vi "remote.Read Dev.Modules.vi"(8 "error in (no error)":errorcluster, 11 "SLSC Remote in":refnum<class "SLSC Interface.lvclass">) -> (0 "error out":errorcluster, 2 "Dev.Modules":refnum<k21>[](array[refnum]), 3 "SLSC Remote out":refnum<class "SLSC Interface.lvclass">)   [LabVIEW 2016, in "SLSC Interface.lvclass"]
uses:
  SLSC Interface Class/SLSC Interface.lvclass
  <vilib>/NI/JSON Support for LabVIEW/JSON Data Classes/JSON Helper/To More Specific Type (Array).vi
  <vilib>/NI/JSON Support for LabVIEW/JSON Data Classes/JSON Array/Index Array (String Value).vi
  <vilib>/NI/JSON Support for LabVIEW/JSON Data Classes/JSON Helper/JSON Helper.lvclass
  <vilib>/NI/JSON Support for LabVIEW/JSON Data Classes/JSON Array/JSON Array.lvclass
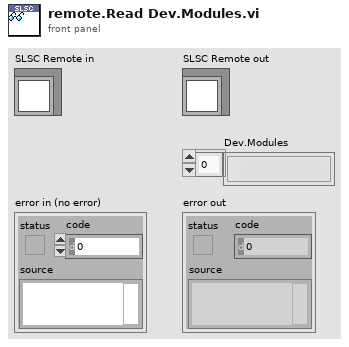
[diagram p1: front panel]
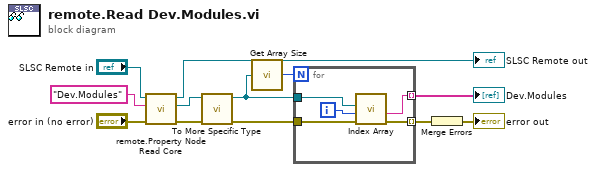
[diagram p0: block diagram]
diagram:
  n1 = call "remote.Property Node Read Core.vi"("error in (no error)"="error in (no error)", "property"="Dev.Modules", "SLSC Remote in"="SLSC Remote in") -> ("error out"=w6:errorcluster, "value"=w2:refnum<class "JSON Null.lvclass">, "SLSC Remote out"=→"SLSC Remote out":refnum<class "SLSC Interface.lvclass">)  [unwired: 6 in]
  n2 = call-poly <vilib>:"To More Specific Type.vi"("error in (no error)"=w6, "JSON Datatype in"=w2) -> ("error out"=w5:errorcluster, "JSON Datatype out"=w1:refnum<class "JSON Array.lvclass">)  [unwired: 8 in]
  n3 = call <vilib>:"Get Array Size.vi"("JSON Array in"=w1) -> ("size(s)"=w8:i32)
  n4 = for {
    N: w8 -> [_]
    tunnel: w1 -> [w17]
    tunnel: [w15] -> w7 mode=indexing
    tunnel: w5 -> [w14]
    tunnel: [w13] -> w4 mode=indexing
    i -> [w16]
    n5 = call-poly <vilib>:"Index Array.vi"("error in (no error)"=w14, "index"=w16, "JSON Array in"=w17) -> ("error out"=w13:errorcluster, "String"=w15:string)  [unwired: 7 in]
  }
  "Dev.Modules" <- w7
  n6 = Merge Errors(w4) -> (→"error out":errorcluster)
